vi "TagDB Refmgr-Register Menu.vi"(7 "menu reference":refnum<k9>, 8 "error in (no error)":errorcluster, 10 "parentURL":string, 11 "TagDB in":T1) -> (0 "error out":errorcluster, 3 "TagDB out":T1)   [LabVIEW 2017, in "TagDB RefManager.lvlib"]
uses:
  TagDB RefManager.lvlib
  <userlib>/_NEVSTOP/TagDB/Typedef/TagDB.ctl
  f04fff1c-0332-4031-a5de-81c0efeec806.vi
  43f95a5c-6252-4fc9-8bb7-ebbefc1e19fa.vi
  <userlib>/_NEVSTOP/TagDB/_Support/DataAccess/data-Write.vi
  <userlib>/_NEVSTOP/TagDB/_Support/DataAccess/TagDB Ref to DVR.vi
  <userlib>/_NEVSTOP/TagDB/_Support/DataAccess/_NameCacher.vi
  <userlib>/_NEVSTOP/TagDB/_Support/DataAccess/_datatypeChecker.vi
  <userlib>/_NEVSTOP/TagDB/_Support/Error/_[error50000]Invalid DB REF.vi
  <vilib>/Utility/Data Type/Get Type Information.vi
  <userlib>/_NEVSTOP/TagDB/TagDB.lvlib
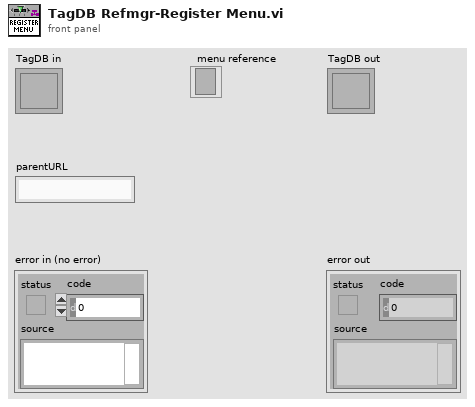
[diagram p1: front panel]
types:
  T1 = typedef "TagDB.lvlib/TagDB.ctl" = refnum<k1>
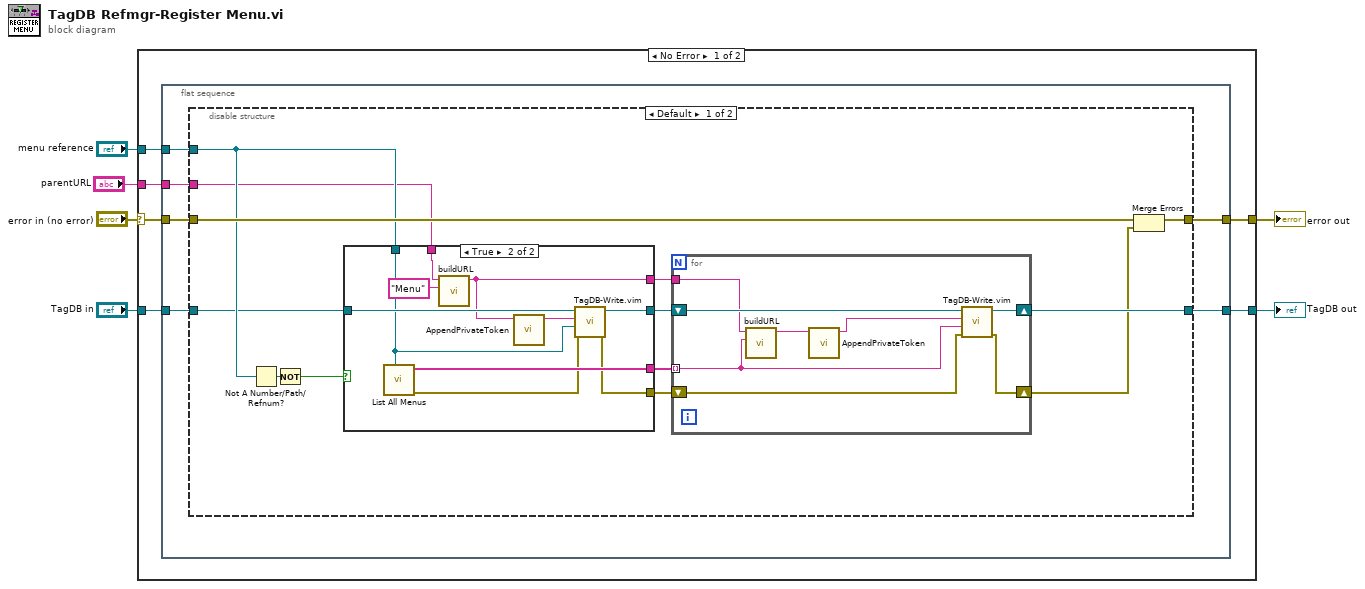
[diagram p0: block diagram]
diagram:
  n1 = case shown="No Error" "error in (no error)" {
    selector: "error in (no error)" -> [w11 w54]
    tunnel: [w12 w54] -> w6
    tunnel: "menu reference" -> [w10 _]
    tunnel: "TagDB in" -> [w8 w53]
    tunnel: [w9 w53] -> w2
    tunnel: "parentURL" -> [w7 _]
    frame No Error {
      n2 = flat-sequence {
        tunnel: [w18] -> w12
        tunnel: w11 -> [w17]
        tunnel: w10 -> [w16]
        tunnel: [w15] -> w9
        tunnel: w8 -> [w13]
        tunnel: w7 -> [w14]
        frame #0 {
          n3 = disable-structure shown="Default" {
            disable-tunnel: [w31 w52] -> w18
            disable-tunnel: w17 -> [w30 w52]
            disable-tunnel: w16 -> [w29 _]
            disable-tunnel: [w26 w51] -> w15
            disable-tunnel: w14 -> [w23 _]
            disable-tunnel: w13 -> [w21 w51]
            frame condition #0 (active) {
              n4 = Not A Number/Path/Refnum?(number/path/refnum=w29) -> (NaN/Path/Refnum?=w28:bool)
              n5 = Not(x=w28) -> (.not. x?=w19:bool)
              n6 = case shown="True" w19 {
                tunnel: w29 -> [_ w41]
                tunnel: [_ w50] -> w27
                tunnel: [_ w43] -> w25
                tunnel: w23 -> [_ w49]
                tunnel: [w40 w46] -> w22
                tunnel: w21 -> [w40 w47]
                tunnel: [_ w42] -> w20
                frame False {
                }
                frame True {
                  n7 = call "List All Menus.vi"("menu reference"=w41) -> ("error in (no error) (dup)"=w44:errorcluster, "Array"=w50:string[])  [unwired: 9 in]
                  n8 = call <userlib>:"buildURL.vi"("DataName"="Menu", "parentURL"=w49) -> ("DataURL"=w42:string)  [unwired: 9 in]
                  n9 = call <userlib>:"AppendPrivateToken.vi"("DataURL"=w42) -> ("String"=w45:string)  [unwired: 10 in]
                  n10 = call "TagDB-Write.vim"("error in (no error)"=w44, "Value"=w41, "tag"=w45, "TagDB"=w47) -> ("error out"=w43:errorcluster, "TagDB(dup)"=w46:T1)  [unwired: 5 in, 1 out]
                }
              }
              n11 = for {
                tunnel: w27 -> [w34] mode=indexing
                shift-right: [w38] -> w26
                shift-left: w22 -> [w39]
                shift-right: [w37] -> w24
                shift-left: w25 -> [w36]
                tunnel: w20 -> [w32]
                n12 = call <userlib>:"buildURL.vi"("DataName"=w34, "parentURL"=w32) -> ("DataURL"=w35:string)  [unwired: 9 in]
                n13 = call <userlib>:"AppendPrivateToken.vi"("DataURL"=w35) -> ("String"=w33:string)  [unwired: 10 in]
                n14 = call "TagDB-Write.vim"("error in (no error)"=w36, "Value"=w34, "tag"=w33, "TagDB"=w39) -> ("error out"=w37:errorcluster, "TagDB(dup)"=w38:T1)  [unwired: 5 in, 1 out]
              }
              n15 = Merge Errors(w30, w24) -> (w31:errorcluster)
            }
            frame condition #1 {
            }
          }
        }
      }
    }
    frame Error {
    }
  }
  "error out" <- w6
  "TagDB out" <- w2
